vi "SpecificErrorHandler.vi"(8 "error in (no error)":errorcluster, 10 "ProcessName":string, 11 "Qbus in":refnum<class "Qbus.lvclass">) -> (0 "error out":errorcluster, 3 "Qbus out":refnum<class "Qbus.lvclass">)   [LabVIEW 2017, in "Loop5.lvlib"]
uses:
  <vilib>/addons/InsightCM/Devices/Shared/Common/DataFlow/test/SpeedBenchmark/Loop5/Loop5.lvlib
  <vilib>/addons/Qbus/Qbus.lvclass
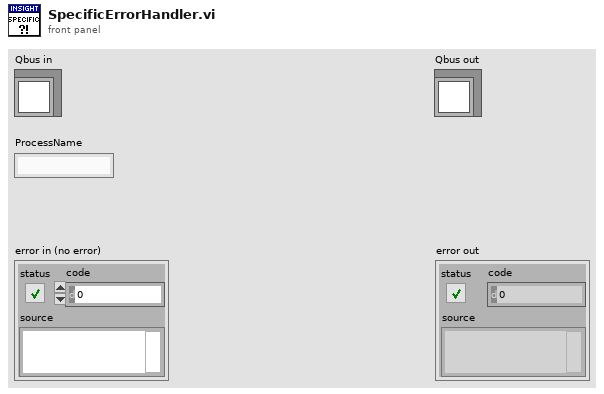
[diagram p1: front panel]
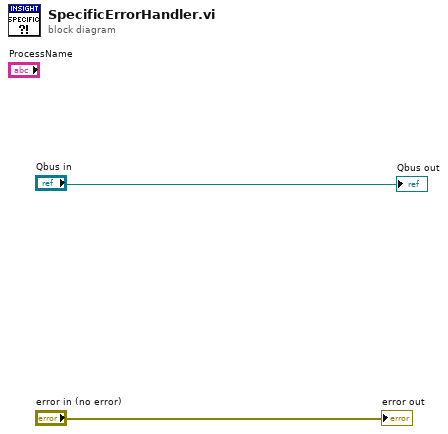
[diagram p0: block diagram]
diagram:
  "error out" <- "error in (no error)"
  "Qbus out" <- "Qbus in"
